vi "FTW-Test-JSON-AddPair.vi"() -> ()   [LabVIEW 2013]
panel:
  out "Error Out":errorcluster
  in  "error In":errorcluster
  in  "Use AddPair for devices?":bool
  in  "Number of Devices":i32=3
  out "Output JSON Object":string
  in  "Number of Items per device":i32=5
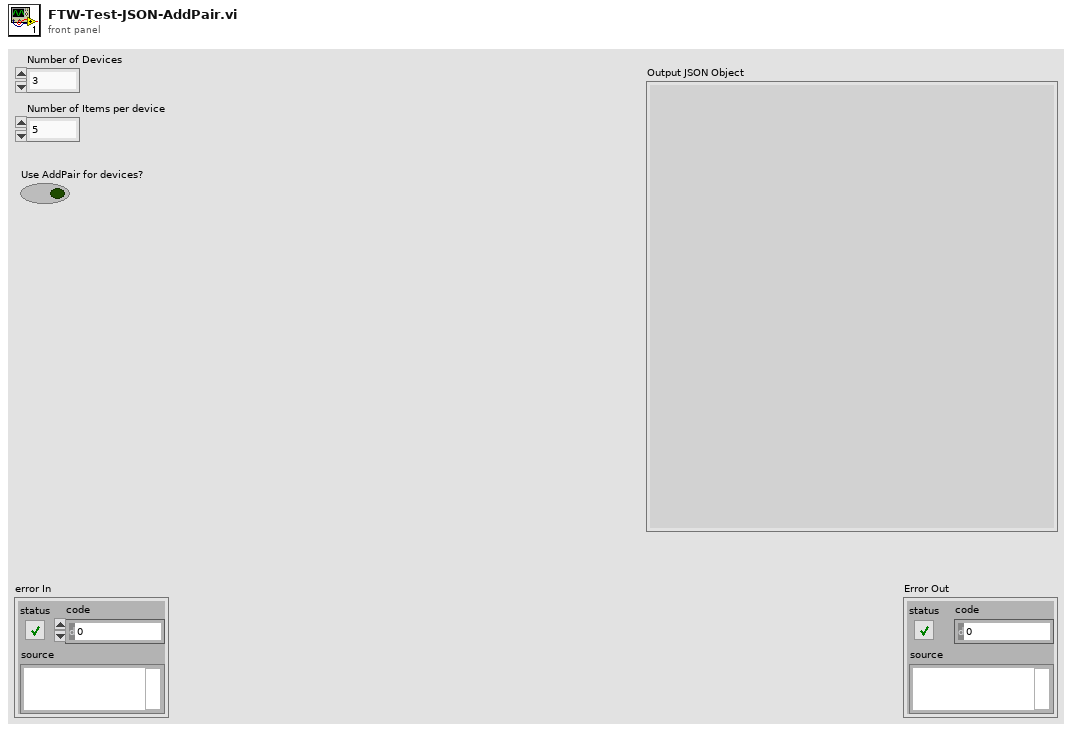
[diagram p1: front panel]
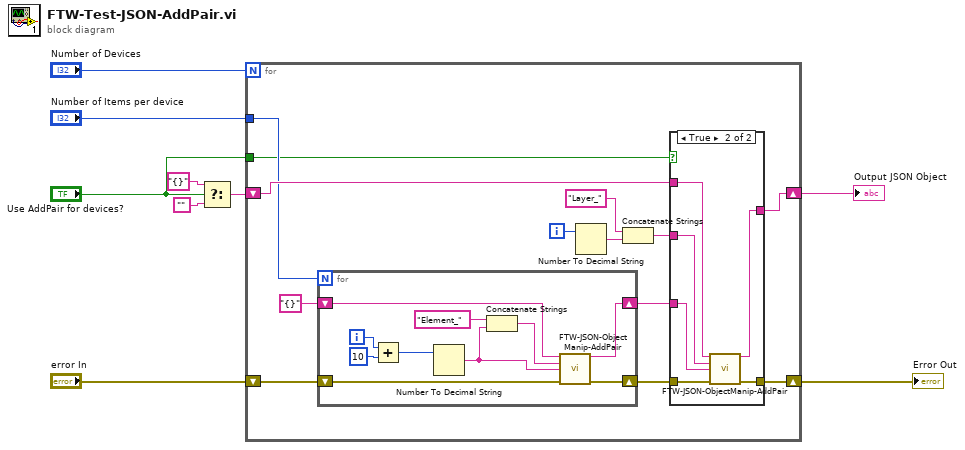
[diagram p0: block diagram]
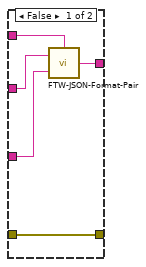
[diagram p2: hidden frame]
diagram:
  n1 = Select(t="{}", s="Use AddPair for devices?", f="" ("Output JSON Object")) -> (s? t:f=w4:string)
  n2 = for {
    N: "Number of Devices" -> [_]
    shift-right: [w18] -> w8
    shift-left: w4 -> [w20]
    tunnel: "Number of Items per device" -> [w17]
    tunnel: "Use AddPair for devices?" -> [w16]
    shift-right: [w14] -> w1
    shift-left: "error In" -> [w13]
    i -> [w22]
    n3 = for {
      N: w17 -> [_]
      shift-right: [w42] -> w19
      shift-left: "{}" ("Output JSON Object") -> [w37]
      shift-right: [w43] -> w15
      shift-left: w13 -> [w38]
      i -> [w41]
      n4 = Add(x=w41, y=10) -> (x+y=w39:i32)
      n5 = Number To Decimal String(number=w39) -> (decimal integer string=w35:string)  [unwired: 1 in]
      n6 = Concatenate Strings("Element_", w35) -> (w34:string)
      n7 = call "FTW-JSON-ObjectManip-AddPair.vi"("Input JSON Object"=w37, "Key"=w34, "Value"=w35, "error in"=w38) -> ("Output JSON Object"=w42:string, "error out"=w43:errorcluster)  [unwired: 10 in]
    }
    n8 = Number To Decimal String(number=w22) -> (decimal integer string=w11:string)  [unwired: 1 in]
    n9 = Concatenate Strings("Layer_", w11) -> (w10:string)
    n10 = case shown="True" w16 {
      tunnel: w20 -> [w27 w30]
      tunnel: w10 -> [w26 w28]
      tunnel: w19 -> [w25 w29]
      tunnel: [w24 w33] -> w18
      tunnel: w15 -> [w23 w32]
      tunnel: [w23 w31] -> w14
      frame False {
        n11 = call "FTW-JSON-Format-Pair.vi"("Prepend to Pair"=w27, "Value"=w25, "Key"=w26) -> ("JSON Pair"=w24:string)
      }
      frame True {
        n12 = call "FTW-JSON-ObjectManip-AddPair.vi"("Input JSON Object"=w30, "Key"=w28, "Value"=w29, "error in"=w32) -> ("Output JSON Object"=w33:string, "error out"=w31:errorcluster)  [unwired: 10 in]
      }
    }
  }
  "Output JSON Object" <- w8
  "Error Out" <- w1
